vi "createCommand.vi"(8 "error in (no error)":errorcluster, 10 "Command":T1, 11 "CommandFactory in":refnum<class "CommandFactory.lvclass">) -> (0 "error out":errorcluster, 2 "command":refnum<class "Command.lvclass">, 3 "CommandFactory out":refnum<class "CommandFactory.lvclass">)   [LabVIEW 2013, in "CommandFactory.lvclass"]
uses:
  CommandFactory.lvclass
  Command/Command.lvclass
  Typedefs/CommandSelector.ctl
  Commands/ClearError/ClearError.lvclass
  Commands/EnableMotion/EnableMotion.lvclass
  Commands/Exit/Exit.lvclass
  Commands/ForceDemand/ForceDemand.lvclass
  Commands/StandBy/StandBy.lvclass
  Commands/Start/Start.lvclass
  Commands/StartAutomatedTest/StartAutomatedTest.lvclass
  Commands/StopAutomatedTest/StopAutomatedTest.lvclass
  Commands/StopMotion/StopMotion.lvclass
  Commands/Update/Update.lvclass
  Typedefs/M2AADTTypedefs.lvlib
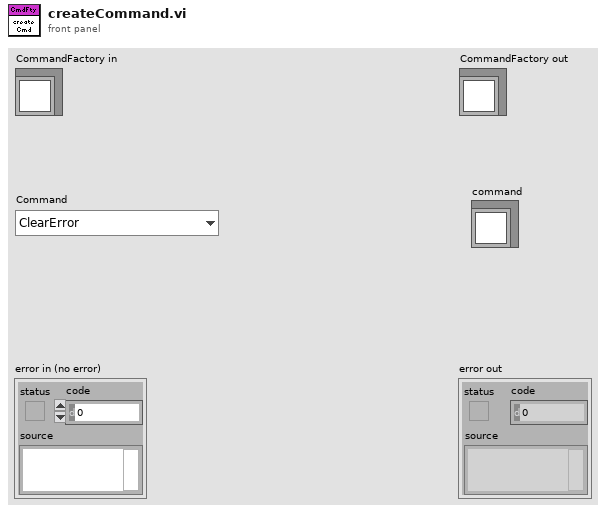
[diagram p1: front panel]
types:
  T1 = typedef "M2AADTTypedefs.lvlib/CommandSelector.ctl" = enum16{"ClearError", "EnableMotion", "Exit", "ForceDemand", "StandBy", "Start", "StartAutomatedTest", "StopAutomatedTest", "StopMotion", "Update"}
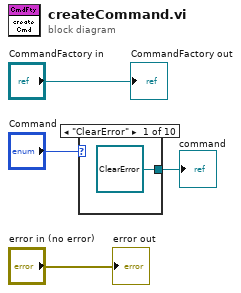
[diagram p0: block diagram]
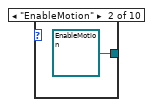
[diagram p2: hidden frame]
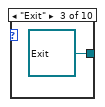
[diagram p3: hidden frame]
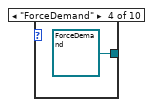
[diagram p4: hidden frame]
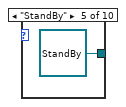
[diagram p5: hidden frame]
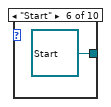
[diagram p6: hidden frame]
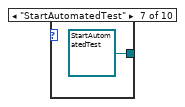
[diagram p7: hidden frame]
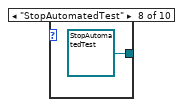
[diagram p8: hidden frame]
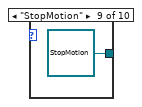
[diagram p9: hidden frame]
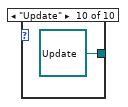
[diagram p10: hidden frame]
diagram:
  n1 = case shown="\"ClearError\"" "Command" {
    tunnel: [refnum<class "ClearError.lvclass"> refnum ("ClearError.lvclass") refnum<class "EnableMotion.lvclass"> refnum ("EnableMotion.lvclass") refnum<class "Exit.lvclass"> refnum ("Exit.lvclass") refnum<class "ForceDemand.lvclass"> refnum ("ForceDemand.lvclass") refnum<class "StandBy.lvclass"> refnum ("StandBy.lvclass") refnum<class "Start.lvclass"> refnum ("Start.lvclass") refnum<class "StartAutomatedTest.lvclass"> refnum ("StartAutomatedTest.lvclass") refnum<class "StopAutomatedTest.lvclass"> refnum ("StopAutomatedTest.lvclass") refnum<class "StopMotion.lvclass"> refnum ("StopMotion.lvclass") refnum<class "Update.lvclass"> refnum ("Update.lvclass")] -> w2
    frame "ClearError" {
    }
    frame "EnableMotion" {
    }
    frame "Exit" {
    }
    frame "ForceDemand" {
    }
    frame "StandBy" {
    }
    frame "Start" {
    }
    frame "StartAutomatedTest" {
    }
    frame "StopAutomatedTest" {
    }
    frame "StopMotion" {
    }
    frame "Update" {
    }
  }
  "command" <- w2
  "error out" <- "error in (no error)"
  "CommandFactory out" <- "CommandFactory in"
